vi "Get All Items By Enumerator.vi"(8 "error in (no error)":errorcluster caption="错误输入（无错误）", 11 "Queue 输入":refnum<class "Queue.lvclass"> caption="DNL_LabVIEW Object in") -> (0 "error out":errorcluster caption="错误输出", 2 "Items":variant[](array[variant]), 3 "Queue 输出":refnum<class "Queue.lvclass"> caption="DNL_LabVIEW Object out")   [LabVIEW 2012, in "Queue.lvclass"]
uses:
  Queue.lvclass
  Enumerator/Enumerator.lvclass
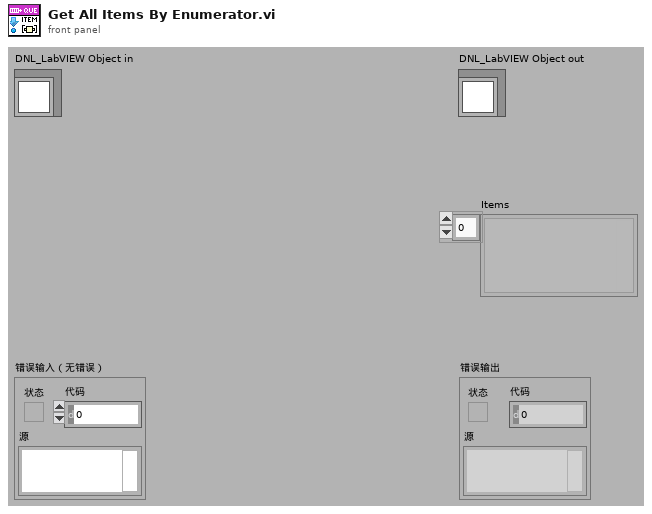
[diagram p1: front panel]
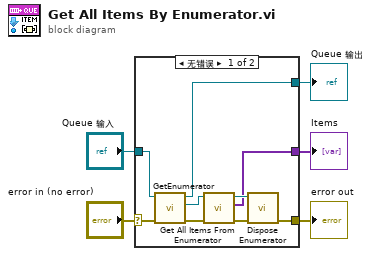
[diagram p0: block diagram]
diagram:
  n1 = case shown="无错误" "error in (no error)" {
    selector: "error in (no error)" -> [w13 w16]
    tunnel: [w7 w16] -> w4
    tunnel: [w11 w15] -> w2
    tunnel: "Queue 输入" -> [w14 w15]
    tunnel: [w6 _] -> w1
    frame No Error {
      n2 = call "GetEnumerator.vi"("error in (no error)"=w13, "Queue 输入"=w14) -> ("error out"=w10:errorcluster, "Enumerator 输出"=w12:refnum<class "Enumerator.lvclass">, "Queue 输出"=w11:refnum<class "Queue.lvclass">)  [unwired: 7 in]
      n3 = call "Get All Items From Enumerator.vi"("error in (no error)"=w10, "Enumerator 输入"=w12) -> ("error out"=w8:errorcluster, "Items"=w6:variant[], "Enumerator 输出"=w9:refnum<class "Enumerator.lvclass">)  [unwired: 7 in]
      n4 = call "Dispose Enumerator.vi"("error in (no error)"=w8, "Enumerator 输入"=w9) -> ("error out"=w7:errorcluster)  [unwired: 8 in, 1 out]
    }
    frame Error {
    }
  }
  "error out" <- w4
  "Queue 输出" <- w2
  "Items" <- w1
